vi "Motion_Gantry Move.vi"(8 "error in (no error)":errorcluster, 10 "Gantry Move Data":T1 {"Z-Position" format="%_7g"; "Y-Position" format="%_7g"; "X-Position" format="%_7g"; "Gantry Velocity" format="%_7g"; "Gantry Accel/Decel" format="%_7g"}, 11 "TCP Connection Refnum in":refnum<k5>) -> (0 "error out":errorcluster, 3 "TCP Connection Refnum (dup)":refnum<k5>)   [LabVIEW 2010]
uses:
  Motion_Gantry Position.ctl
  Motion_Coils Typedef.ctl
  Motion_Registers Typedef.ctl
  <vilib>/NI Modbus.llb/MB Ethernet Master Query Write Multiple Registers (poly).vi
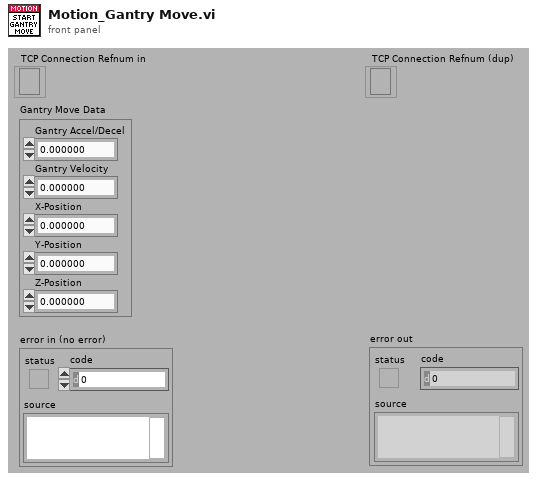
[diagram p1: front panel]
types:
  T1 = typedef "Motion_Gantry Position.ctl" = cluster{"Gantry Accel/Decel":dbl, "Gantry Velocity":dbl, "X-Position":dbl, "Y-Position":dbl, "Z-Position":dbl}
  T2 = typedef "Motion_Coils Typedef.ctl" = u16
  T3 = typedef "Motion_Registers Typedef.ctl" = u16
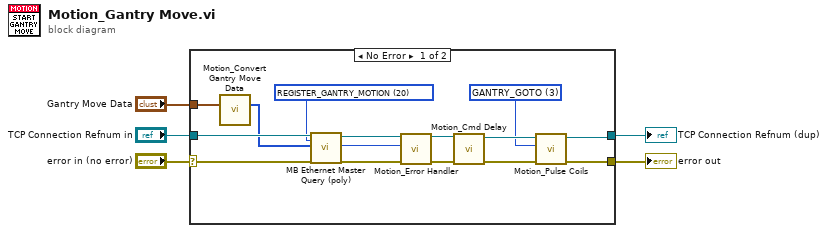
[diagram p0: block diagram]
diagram:
  n1 = case shown="No Error" "error in (no error)" {
    selector: "error in (no error)" -> [w19 w21]
    tunnel: "TCP Connection Refnum in" -> [w20 w22]
    tunnel: [w8 w22] -> w4
    tunnel: "Gantry Move Data" -> [w18 _]
    tunnel: [w7 w21] -> w1
    frame No Error {
      w6 = T2 3 items=["GANTRY_ENABLE"=1, "GANTRY_GOTO"=3] ("Coils")
      w16 = T3 20 items=["REGISTER_GANTRY_MOTION"=20] ("Registers")
      n2 = call "Motion_Convert Gantry Move Data.vi"("Gantry Move Data"=w18) -> ("Gantry Move data"=w17:u16[])  [unwired: 14 in]
      n3 = call-poly <vilib>:"MB Ethernet Master Query (poly).vi"("TCP Connection Refnum in"=w20, "Starting Address"=w16, "Registers"=w17, "error in"=w19) -> ("TCP Connection Refnum (dup)"=w13:refnum<k5>, "Exception Code"=w14:u8, "error out"=w15:errorcluster)  [unwired: 13 in]
      n4 = call "Motion_Error Handler.vi"("error in (no error)"=w15, "Exception Code"=w14, "TCP Connection Refnum in"=w13) -> ("error out"=w11:errorcluster, "TCP Connection Refnum (dup)"=w12:refnum<k5>)  [unwired: 7 in]
      n5 = call "Motion_Cmd Delay.vi"("error in"=w11, "TCP Connection Refnum"=w12) -> ("error out"=w9:errorcluster, "TCP Connection Refnum (dup)"=w10:refnum<k5>)  [unwired: 8 in]
      n6 = call "Motion_Pulse Coils.vi"("error in"=w9, "Pulse Coil"=w6, "TCP refnum"=w10) -> ("error out"=w7:errorcluster, "TCP refnum dup"=w8:refnum<k5>)  [unwired: 7 in]
    }
    frame Error {
    }
  }
  "TCP Connection Refnum (dup)" <- w4
  "error out" <- w1
